vi "Render Template.vi"(9 "Variables in":map{string, string[]}(c390), 10 "Endpoint":string, 11 "Request":T1) -> (2 "Content-Type":string, 3 "Content out":string)   [LabVIEW 2021, in "HttpServer.lvlib"]
uses:
  HttpServer.lvlib
  TypeDefs/Request.ctl
  TypeDefs/Action.ctl
panel:
  out "result string":string
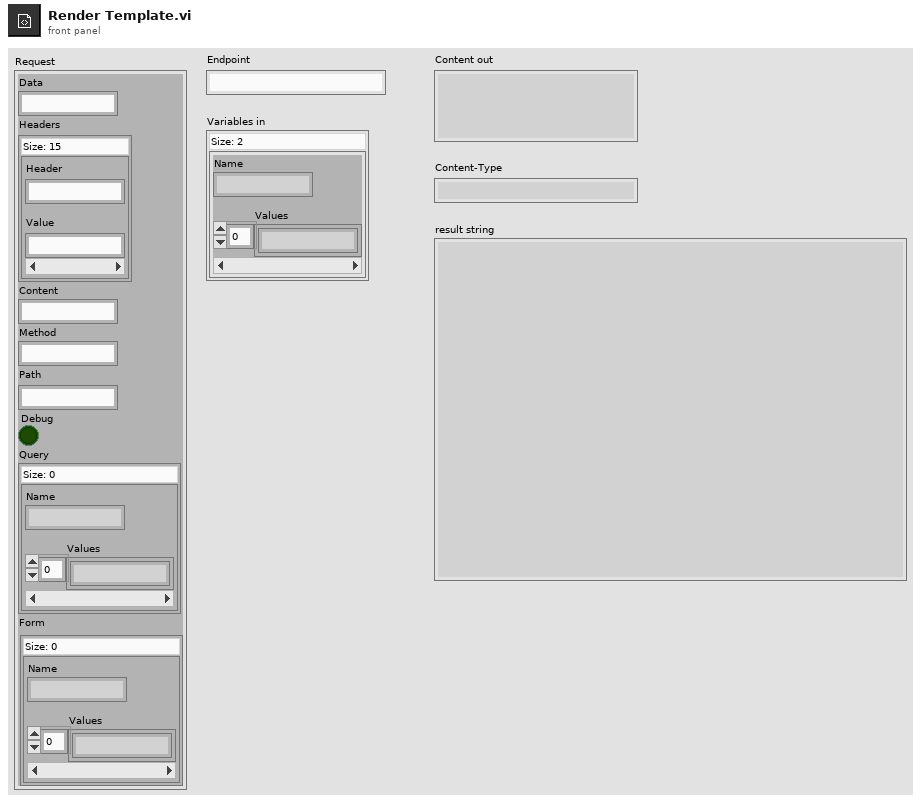
[diagram p1: front panel]
types:
  T1 = typedef "HttpServer.lvlib/Request.ctl" = cluster{"Data":string, "Headers":map{string, string}, "Content":string, "Method":string, "Path":string, "Debug":bool, "Query":map{string, string[]}, "Form":map{string, string[]}}
  T2 = typedef "HttpServer.lvlib/Action.ctl" = enum8{"noop", "add", "get", "set", "remove"}
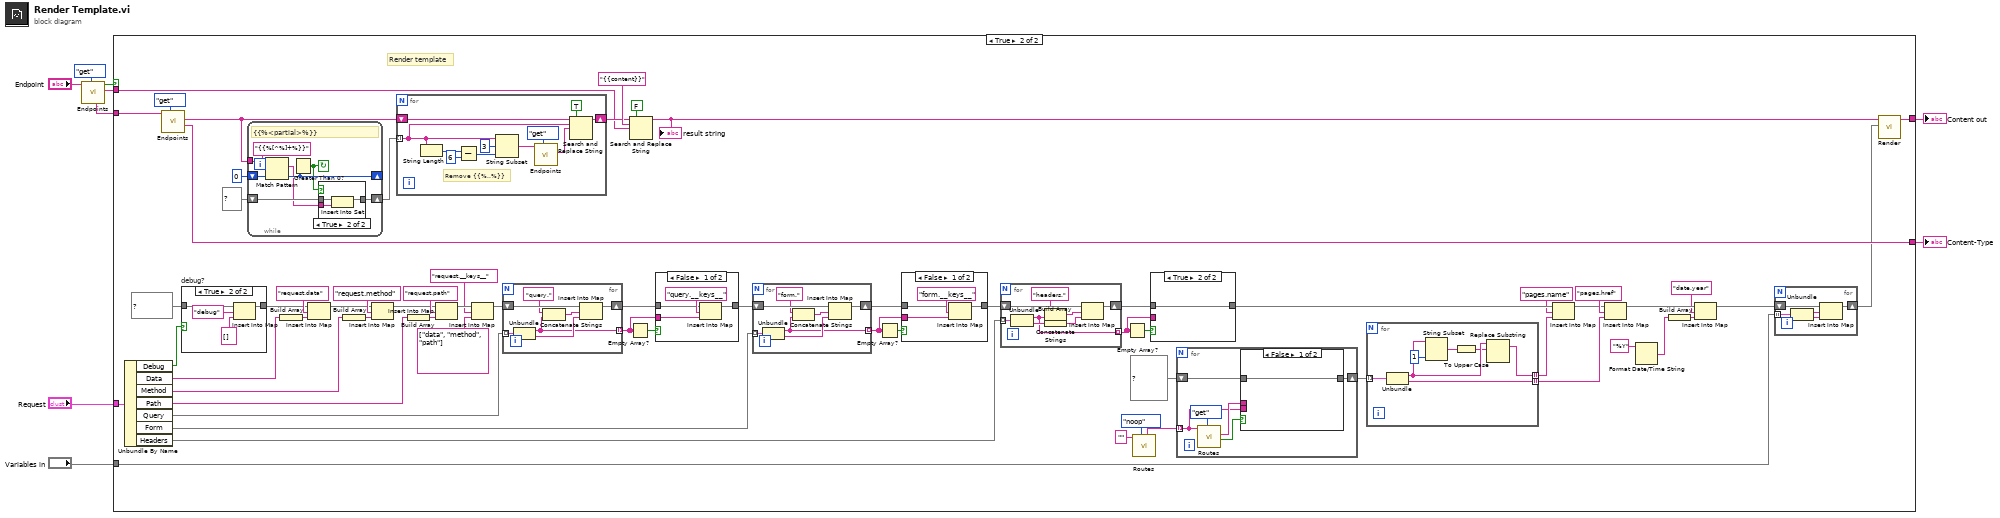
[diagram p0: block diagram]
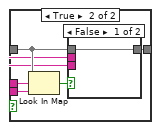
[diagram p3: hidden frame]
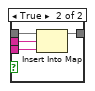
[diagram p4: hidden frame]
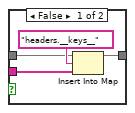
[diagram p5: hidden frame]
diagram:
  n1 = call "Endpoints.vi"("Action"=Action."get", "Endpoint"="Endpoint") -> ("Content out"=w4:string, "Found?"=w1:bool, "Template out"=w5:string)  [unwired: 4 in, 3 out]
  n2 = case shown="True" w1 {
    tunnel: [_ w74] -> w9
    tunnel: [_ w69] -> w8
    tunnel: "Request" -> [_ w68]
    tunnel: w5 -> [_ w67]
    tunnel: w4 -> [_ w28]
    tunnel: "Variables in" -> [_ w34]
    frame False {
    }
    frame True {
      # "Render template"
      n3 = Unbundle By Name(w68) -> ("Debug"=w65:bool, "Data"=w66:string, "Method"=w58:string, "Path"=w54:string, "Query"=w52:map{string, string[]}, "Form"=w41:map{string, string[]}, "Headers"=w51:map{string, string})
      n4 = call "Endpoints.vi"("Action"=Action."get", "Endpoint"=w67) -> ("Content-Type out"=w69:string, "Content out"=w33:string)  [unwired: 4 in, 4 out]
      n5 = case "debug?" shown="True" w65 {
        tunnel: map{string, string[]} {} ("Keys") -> [w159 w163]
        tunnel: [w159 w162] -> w63
        frame False {
        }
        frame True {
          n6 = Insert Into Map(map in=w163, key="debug", value=string[] [] ("Values")) -> (map out=w162:map{string, string[]})  [unwired: 2 out]
        }
      }
      n7 = while {
        tunnel: w33 -> [w143]
        shift-right: [w141] -> _
        shift-left: 0 ("offset (0)") -> [w142]
        shift-right: [w138] -> w71
        shift-left: set{string} {} ("Size: 0") -> [w139]
        stop <- w137 continue-if-true
        # "{{%<partial>%}}"
        n8 = Match Pattern(string=w143, regular expression="{{%[^%]+%}}", offset (0)=w142) -> (match substring=w136:string, offset past match=w141:i32)  [unwired: 2 out]
        n9 = Greater Than 0?(x=w141) -> (x > 0?=w137:bool)
        n10 = case shown="True" w137 {
          tunnel: w139 -> [w144 w147]
          tunnel: [w144 w146] -> w138
          tunnel: w136 -> [_ w145]
          frame False {
          }
          frame True {
            n11 = Insert Into Set(10:w145, 11:w147) -> (3:w146:set{string})  [unwired: 1 out]
          }
        }
      }
      n12 = Build Array(w66) -> (w62:string[])
      n13 = Insert Into Map(map in=w63, key="request.data", value=w62) -> (map out=w59:map{string, string[]})  [unwired: 2 out]
      n14 = Build Array(w58) -> (w61:string[])
      n15 = Insert Into Map(map in=w59, key="request.method", value=w61) -> (map out=w55:map{string, string[]})  [unwired: 2 out]
      n16 = for {
        tunnel: w71 -> [w148] mode=indexing
        shift-right: [w155] -> w30
        shift-left: w33 -> [w157]
        # "Remove {{%..%}}"
        n17 = String Length(string=w148) -> (length=w152:i32)
        n18 = Subtract(x=w152, y=6) -> (x-y=w150:i32)
        n19 = String Subset(string=w148, offset (0)=3, length (rest)=w150) -> (substring=w149:string)
        n20 = call "Endpoints.vi"("Action"=Action."get", "Endpoint"=w149) -> ("Content out"=w154:string)  [unwired: 4 in, 5 out]
        n21 = Search and Replace String(replace all?=TRUE ("replace all? (F)"), input string=w157, search string=w148, replace string=w154) -> (result string=w155:string)  [unwired: 4 in, 3 out]
      }
      n22 = Build Array(w54) -> (w56:string[])
      n23 = Insert Into Map(map in=w55, key="request.path", value=w56) -> (map out=w53:map{string, string[]})  [unwired: 2 out]
      n24 = Insert Into Map(map in=w53, key="request.__keys__", value=string[] ["data", "method", "path"]) -> (map out=w50:map{string, string[]})  [unwired: 2 out]
      n25 = for {
        shift-right: [w134] -> w47
        shift-left: w50 -> [w135]
        tunnel: w52 -> [w133] mode=indexing
        tunnel: [w129] -> w46 mode=indexing
        n26 = Unbundle(w133) -> ("Name"=w129:string, "Values"=w130:string[])
        n27 = Concatenate Strings("query." ("string"), w129) -> (w131:string)
        n28 = Insert Into Map(map in=w135, key=w131, value=w130) -> (map out=w134:map{string, string[]})  [unwired: 2 out]
      }
      n29 = Empty Array?(array=w46) -> (empty?=w45:bool)
      n30 = Search and Replace String(replace all?=FALSE ("replace all? (F)"), input string=w30, search string="{{content}}", replace string=w28) -> (result string=w29:string)  [unwired: 4 in, 3 out]
      "result string" <- w29
      n31 = case shown="False" w45 {
        tunnel: w47 -> [w118 w120]
        tunnel: w46 -> [w117 _]
        tunnel: [w116 w120] -> w40
        frame False {
          n32 = Insert Into Map(map in=w118, key="query.__keys__", value=w117) -> (map out=w116:map{string, string[]})  [unwired: 2 out]
        }
        frame True {
        }
      }
      n33 = for {
        shift-right: [w114] -> w42
        shift-left: w40 -> [w115]
        tunnel: w41 -> [w113] mode=indexing
        tunnel: [w109] -> w43 mode=indexing
        n34 = Unbundle(w113) -> ("Name"=w109:string, "Values"=w110:string[])
        n35 = Concatenate Strings("form." ("string"), w109) -> (w111:string)
        n36 = Insert Into Map(map in=w115, key=w111, value=w110) -> (map out=w114:map{string, string[]})  [unwired: 2 out]
      }
      n37 = Empty Array?(array=w43) -> (empty?=w44:bool)
      n38 = case shown="False" w44 {
        tunnel: w42 -> [w106 w108]
        tunnel: w43 -> [w105 _]
        tunnel: [w104 w108] -> w39
        frame False {
          n39 = Insert Into Map(map in=w106, key="form.__keys__", value=w105) -> (map out=w104:map{string, string[]})  [unwired: 2 out]
        }
        frame True {
        }
      }
      n40 = for {
        shift-right: [w127] -> w36
        shift-left: w39 -> [w128]
        tunnel: w51 -> [w126] mode=indexing
        tunnel: [w121] -> w35 mode=indexing
        n41 = Unbundle(w126) -> ("Header"=w121:string, "Value"=w123:string)
        n42 = Concatenate Strings("headers." ("string"), w121) -> (w124:string)
        n43 = Build Array(w123) -> (w122:string[])
        n44 = Insert Into Map(map in=w128, key=w124, value=w122) -> (map out=w127:map{string, string[]})  [unwired: 2 out]
      }
      n45 = Empty Array?(array=w35) -> (empty?=w37:bool)
      n46 = call "Routes.vi"("Action"=Action."noop", "Path"="") -> ("Paths"=w23:string[])  [unwired: 6 in, 3 out]
      n47 = case shown="True" w37 {
        tunnel: w36 -> [w101 w103]
        tunnel: w35 -> [w100 _]
        tunnel: [w99 w103] -> w27
        frame False {
          n48 = Insert Into Map(map in=w101, key="headers.__keys__", value=w100) -> (map out=w99:map{string, string[]})  [unwired: 2 out]
        }
        frame True {
        }
      }
      n49 = for {
        tunnel: w23 -> [w83] mode=indexing
        shift-right: [w86] -> w21
        shift-left: map{string, string} {} ("Map") -> [w85]
        n50 = call "Routes.vi"("Action"=Action."get", "Path"=w83) -> ("Is Navbar Page?"=w82:bool, "Endpoint out"=w84:string)  [unwired: 6 in, 2 out]
        n51 = case shown="False" w82 {
          tunnel: [w88 w93] -> w86
          tunnel: w85 -> [w88 w92]
          tunnel: w84 -> [_ w91]
          tunnel: w83 -> [_ w89]
          frame False {
          }
          frame True {
            n52 = Look In Map(map=w92, key=w91, default value=w89) -> (key not found?=w90:bool)  [unwired: 1 out]
            n53 = case shown="False" w90 {
              tunnel: [w94 w98] -> w93
              tunnel: w92 -> [w94 w97]
              tunnel: w91 -> [_ w96]
              tunnel: w89 -> [_ w95]
              frame False {
              }
              frame True {
                n54 = Insert Into Map(map in=w97, key=w96, value=w95) -> (map out=w98:map{string, string})  [unwired: 2 out]
              }
            }
          }
        }
      }
      n55 = for {
        tunnel: w21 -> [w81] mode=indexing
        tunnel: [w76] -> w20 mode=indexing
        tunnel: [w80] -> w16 mode=indexing
        n56 = Unbundle(w81) -> ("Endpoint"=w77:string, "Path"=w80:string)
        n57 = String Subset(string=w77, length (rest)=1 ("length (rest)")) -> (substring=w78:string)  [unwired: 1 in]
        n58 = To Upper Case(1:w78) -> (0:w75:string)
        n59 = Replace Substring(4:w75, 5:w77) -> (1:w76:string)  [unwired: 2 in, 1 out]
      }
      n60 = Insert Into Map(map in=w27, key="pages.name" ("string"), value=w20) -> (map out=w17:map{string, string[]})  [unwired: 2 out]
      n61 = Insert Into Map(map in=w17, key="pages.href" ("string"), value=w16) -> (map out=w15:map{string, string[]})  [unwired: 2 out]
      n62 = Format Date/Time String(time format string (%c)="%Y") -> (date/time string=w11:string)  [unwired: 2 in]
      n63 = Build Array(w11) -> (w10:string[])
      n64 = Insert Into Map(map in=w15, key="date.year", value=w10) -> (map out=w14:map{string, string[]})  [unwired: 2 out]
      n65 = for {
        shift-right: [w167] -> w26
        shift-left: w14 -> [w168]
        tunnel: w34 -> [w166] mode=indexing
        n66 = Unbundle(w166) -> ("Name"=w164:string, "Values"=w165:string[])
        n67 = Insert Into Map(map in=w168, key=w164, value=w165) -> (map out=w167:map{string, string[]})  [unwired: 2 out]
      }
      n68 = call "Render.vi"("Keys"=w26, "Content in"=w29) -> ("Content out"=w74:string)  [unwired: 9 in]
    }
  }
  "Content out" <- w9
  "Content-Type" <- w8
